vi "DEVICE_CONNECT_n.vi"(2 "execute":bool, 11 "error in (no error)":errorcluster) -> (4 "function return":string, 8 "uLPtr":u32[](array[numeric]), 10 "serial no":string, 15 "error out":errorcluster)   [LabVIEW 2017, in "ZBOX_IS.lvlib"]
uses:
  ZBOX_IS.lvlib
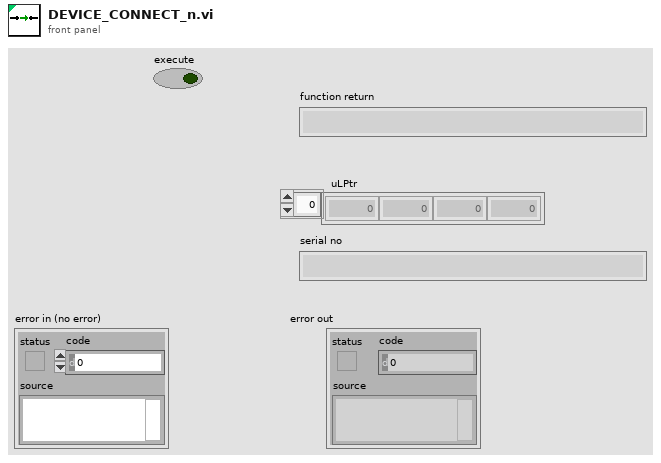
[diagram p1: front panel]
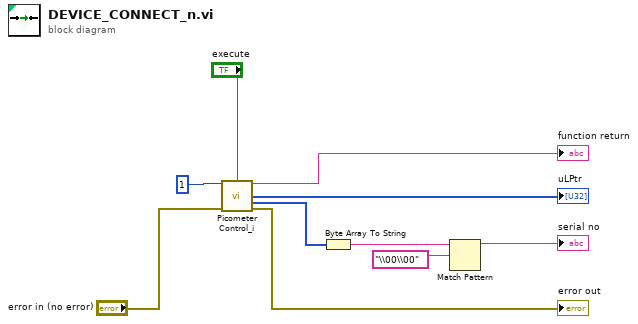
[diagram p0: block diagram]
diagram:
  n1 = call "Picometer Control_i.vi"("Cmd"=u8 1, "execute"="execute", "error in (no error)"="error in (no error)") -> ("function return"=→"function return":string, "uLPtr"=→"uLPtr":u32[], "BytePtr"=w5:u8[], "error out"=→"error out":errorcluster)  [unwired: 8 in, 1 out]
  n2 = Byte Array To String(unsigned byte array=w5) -> (string=w2:string)
  n3 = Match Pattern(string=w2, regular expression="\\00\\00") -> (before substring=→"serial no":string)  [unwired: 1 in, 3 out]
